vi "Init.vi"(8 "error in (no error)":errorcluster, 10 "Channel Index":i32, 11 "Group":refnum<class "Group.lvclass">) -> (0 "error out":errorcluster, 3 "Channel out":refnum<class "Channel.lvclass">)   [LabVIEW 2020, in "Vecto.lvlib" / "Channel.lvclass"]
uses:
  Channel.lvclass
  Group/Group.lvclass
  Channel.lvclass/Channel.ctl
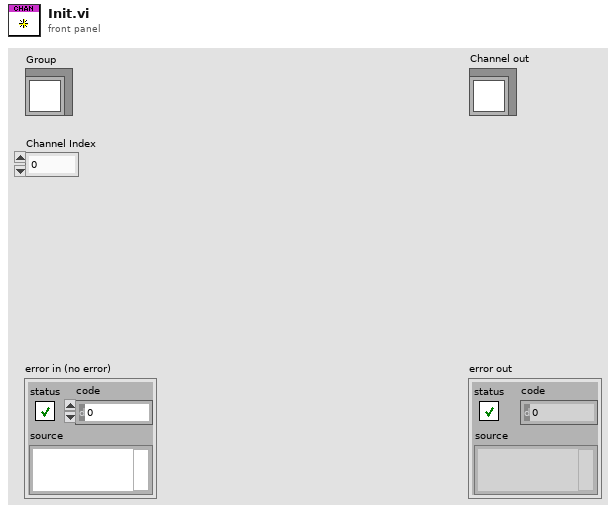
[diagram p1: front panel]
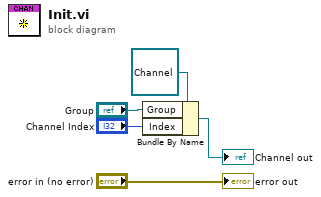
[diagram p0: block diagram]
diagram:
  n1 = Bundle By Name(cluster=refnum<class "Channel.lvclass"> refnum ("Channel in"), "Group"="Group", "Index"="Channel Index") -> (→"Channel out":refnum<class "Channel.lvclass">)
  "error out" <- "error in (no error)"
